vi "PROJETTTT.vi"(0 "Numérique":i32, 1 "stop":bool) -> (2 "Nb cycles":dbl, 3 "Produits Finis":dbl, 4 "Produits defectueux":dbl)   [LabVIEW 2024]
uses:
  lcanneta.ctl
  selector.ctl
panel:
  in  "Bouton OK":bool
  out "Capteur de présence":bool
  out "Début course":bool
  out "Fin de course":bool
  out "Booléen":bool
  in  "RESET":bool
  in  "Selector":T1
  out "Glissière":T2 scale=0.0..100.0
  # "STOP"
  # "START"
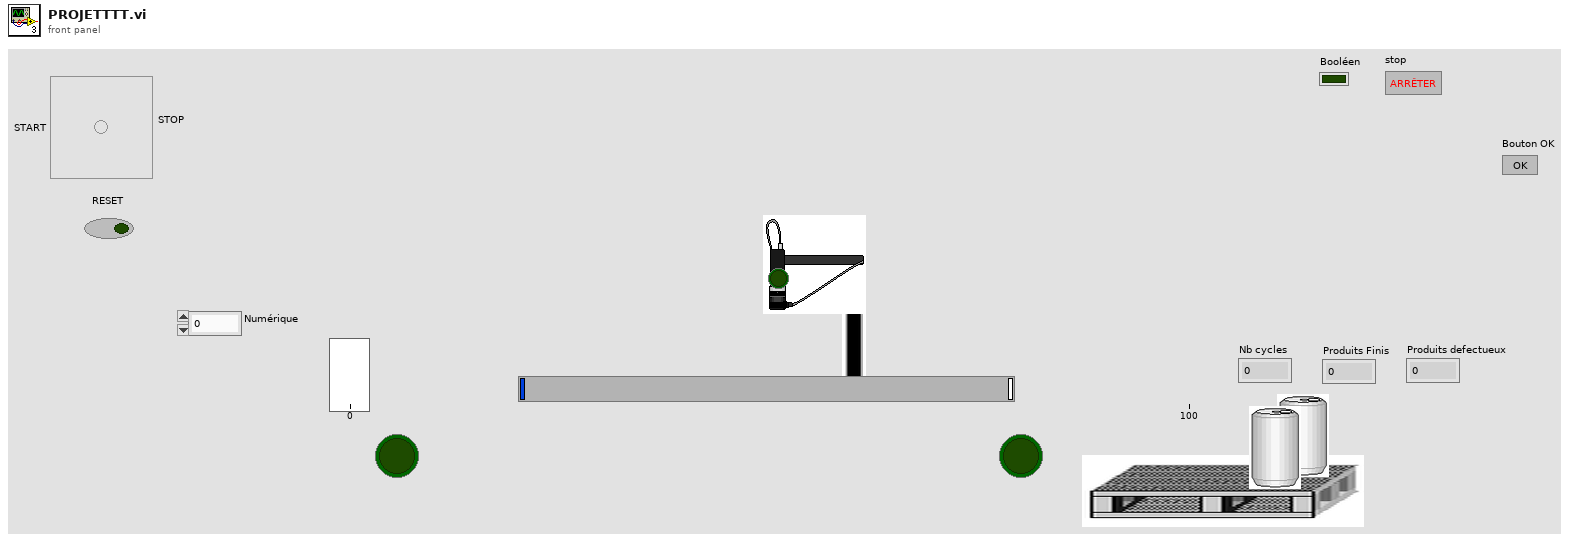
[diagram p1: front panel]
types:
  T1 = typedef "selector.ctl" = bool
  T2 = typedef "lcanneta.ctl" = dbl
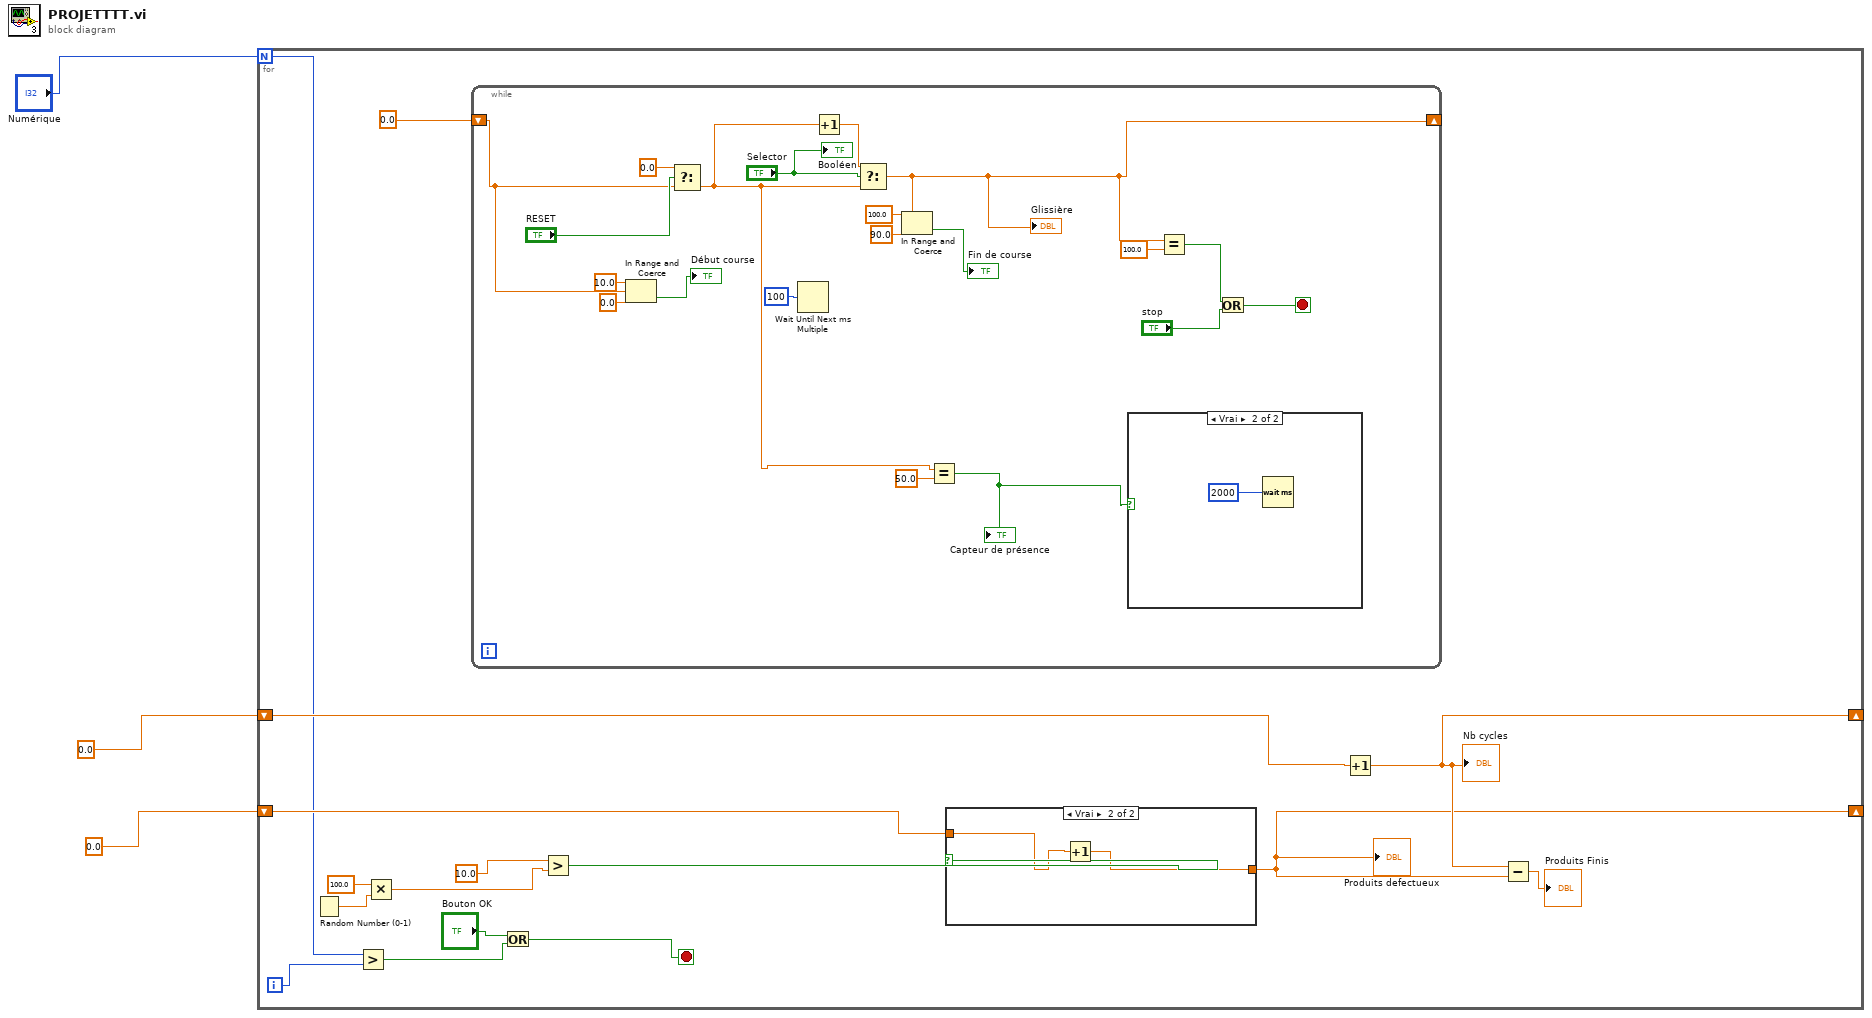
[diagram p0: block diagram]
diagram:
  n1 = for {
    N: "Numérique" -> [w8]
    shift-right: [w10] -> _
    shift-left: 0.0 ("x") -> [w18]
    shift-right: [w9] -> _
    shift-left: 0.0 ("x") -> [w12]
    i -> [w7]
    stop <- w4 stop-if-true
    n2 = Random Number (0-1)() -> (number: 0 to 1=w17:dbl)
    n3 = Greater?(x=w8, y=w7) -> (0:w5:bool)
    n4 = Multiply(x=100.0, y=w17) -> (x*y=w15:dbl)
    n5 = while {
      shift-right: [w24] -> _
      shift-left: 0.0 -> [w32]
      stop <- w27 stop-if-true
      n6 = In Range and Coerce(upper limit=10.0 ("limite supérieure"), x=w32, lower limit=0.0 ("limite inférieure")) -> (In Range?=→"Début course":bool)  [unwired: 1 out]
      n7 = Select(t=0.0 ("cas vrai"), s="RESET", f=w32) -> (s? t:f=w29:dbl)
      n8 = Wait Until Next ms Multiple(millisecond multiple=u32 100 ("n millisecondes")) -> ()  [unwired: 1 out]
      n9 = Increment(x=w29) -> (x+1=w40:dbl)
      n10 = Select(t=w40, s="Selector", f=w29) -> (s? t:f=w24:dbl)
      "Glissière" <- w24
      n11 = In Range and Coerce(upper limit=100.0 ("limite supérieure"), x=w24, lower limit=90.0 ("limite inférieure")) -> (In Range?=→"Fin de course":bool)  [unwired: 1 out]
      n12 = Equal?(x=w29, y=50.0) -> (x = y?=w28:bool)
      "Capteur de présence" <- w28
      n13 = case shown="Vrai" w28 {
        frame False {
        }
        frame True {
          n14 = Wait (ms)(milliseconds to wait=u32 2000 ("valeur de l'horloge en ms")) -> ()  [unwired: 1 out]
        }
      }
      n15 = Equal?(x=w24, y=100.0) -> (x = y?=w23:bool)
      n16 = Or(x=w23, y="stop") -> (x .or. y?=w27:bool)
      "Booléen" <- "Selector"
    }
    n17 = Or(x="Bouton OK", y=w5) -> (x .or. y?=w4:bool)
    n18 = Greater?(x=10.0, y=w15) -> (0:w13:bool)
    n19 = case shown="Vrai" w13 {
      tunnel: w12 -> [w20 w22]
      tunnel: [w20 w21] -> w9
      frame False {
      }
      frame True {
        n20 = Increment(x=w22) -> (x+1=w21:dbl)
      }
    }
    "Produits defectueux" <- w9
    n21 = Increment(x=w18) -> (x+1=w10:dbl)
    "Nb cycles" <- w10
    n22 = Subtract(x=w10, y=w9) -> (x-y=→"Produits Finis":dbl)
  }
